vi "KeyBdReader.vi"(8 "error in (no error)":errorcluster) -> (0 "error out":errorcluster)   [LabVIEW 2014]
uses:
  c_InstructionEnum.ctl
  g_Stop.vi
  <vilib>/Utility/inputDevices.llb/keyboardAcquire.vi
  g_CommandParam.vi
  <vilib>/Utility/inputDevices.llb/closeKeyboard.vi
  c_PlatePosEnum.ctl
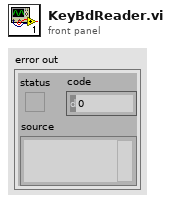
[diagram p1: front panel]
types:
  T1 = typedef "c_InstructionEnum.ctl" = enum16{"Move Absolute", "Increment", "Move Home", "Motion Kill", "Move Plate", "Set Stepsize", "Query Position"}
  T2 = typedef "c_PlatePosEnum.ctl" = enum16{"Contact", "Seperate"}
  T3 = enum16{"0", "1", "2", "3", "4", "5", "6", "7", "8", "9", "A", "B", "C", "D", "E", "F", "G", "H", "I", "J", "K", "L", "M", "N", "O", "P", "Q", "R", "S", "T", "U", "V", "W", "X", "Y", "Z", "F1", "F2", "F3", "F4", "F5", "F6", "F7", "F8", "F9", "F10", "F11", "F12", "F13", "F14", "F15", "ADD", "BACK", "BACKSLASH", "CAPITAL", "COMMA", "DECIMAL", "DELETE", "DIVIDE", "DOWN", "END", "EQUALS", "ESCAPE", "GRAVE (`)", "HOME", "INSERT", "LBRACKET", "LCONTROL", "LEFT", "L ALT", "LSHIFT", "LWIN", "MINUS", "MULTIPLY", "NEXT", "NUMLOCK", "NUMPAD_0", "NUMPAD_1", "NUMPAD_2", "NUMPAD_3", "NUMPAD_4", "NUMPAD_5", "NUMPAD_6", "NUMPAD_7", "NUMPAD_8", "NUMPAD_9", "PAUSE", "PERIOD", "PRIOR (PG UP)", "RBRACKET", "RCONTROL", "RETURN", "RIGHT", "R ALT", "RSHIFT", "RWIN", "SCROLL", "SEMICOLON", "SLASH", "SPACE", "SUBTRACT", "TAB", "UP", "ENTER (num pad)", "' (quote)"}[]
  T4 = enum16{"0", "1", "2", "3", "4", "5", "6", "7", "8", "9", "A", "B", "C", "D", "E", "F", "G", "H", "I", "J", "K", "L", "M", "N", "O", "P", "Q", "R", "S", "T", "U", "V", "W", "X", "Y", "Z", "F1", "F2", "F3", "F4", "F5", "F6", "F7", "F8", "F9", "F10", "F11", "F12", "F13", "F14", "F15", "ADD", "BACK", "BACKSLASH", "CAPITAL", "COMMA", "DECIMAL", "DELETE", "DIVIDE", "DOWN", "END", "EQUALS", "ESCAPE", "GRAVE (`)", "HOME", "INSERT", "LBRACKET", "LCONTROL", "LEFT", "L ALT", "LSHIFT", "LWIN", "MINUS", "MULTIPLY", "NEXT", "NUMLOCK", "NUMPAD_0", "NUMPAD_1", "NUMPAD_2", "NUMPAD_3", "NUMPAD_4", "NUMPAD_5", "NUMPAD_6", "NUMPAD_7", "NUMPAD_8", "NUMPAD_9", "PAUSE", "PERIOD", "PRIOR (PG UP)", "RBRACKET", "RCONTROL", "RETURN", "RIGHT", "R ALT", "RSHIFT", "RWIN", "SCROLL", "SEMICOLON", "SLASH", "SPACE", "SUBTRACT", "TAB", "UP", "ENTER (num pad)", "' (quote)"}
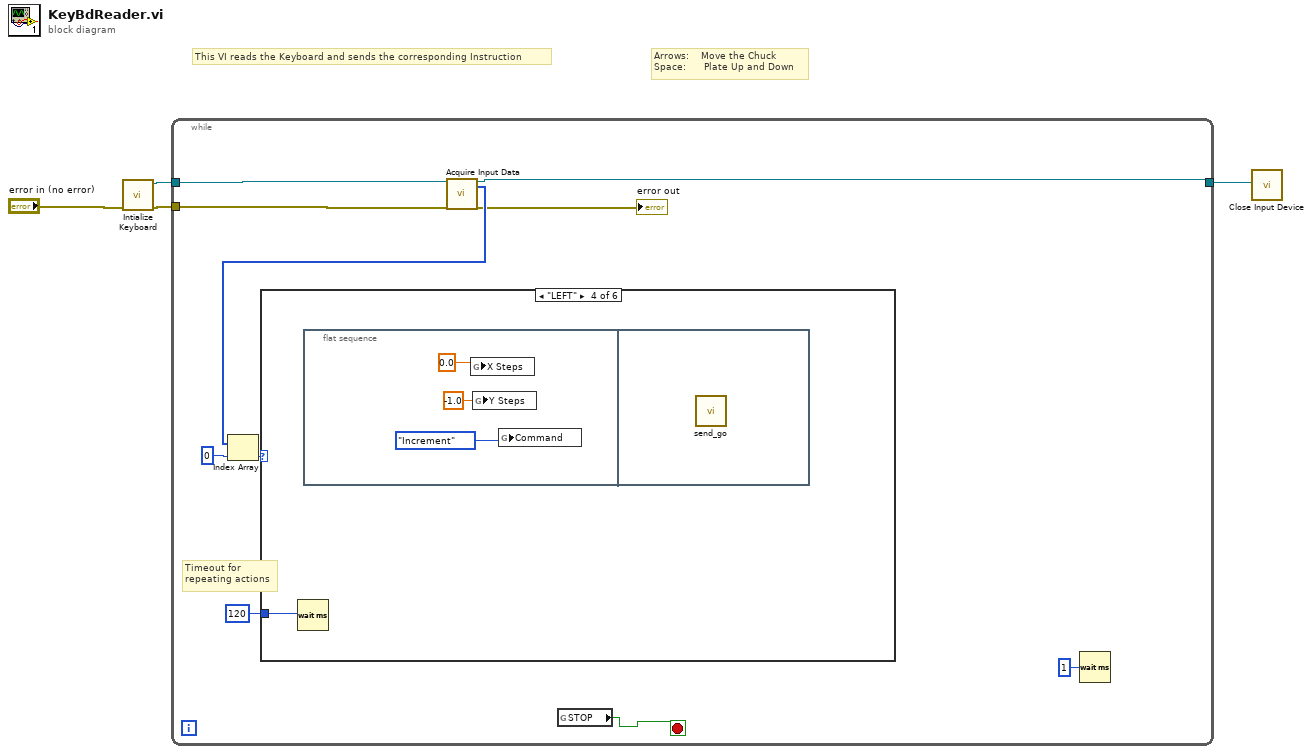
[diagram p0: block diagram]
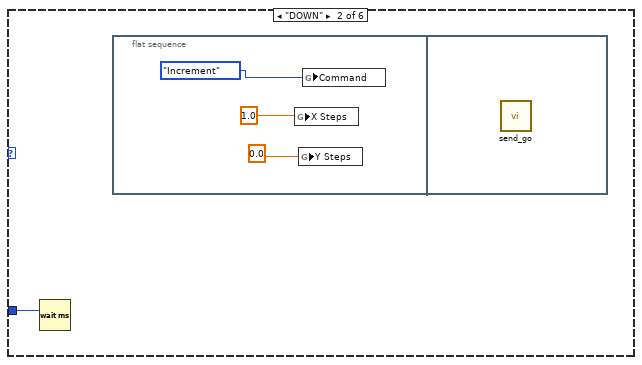
[diagram p3: hidden frame]
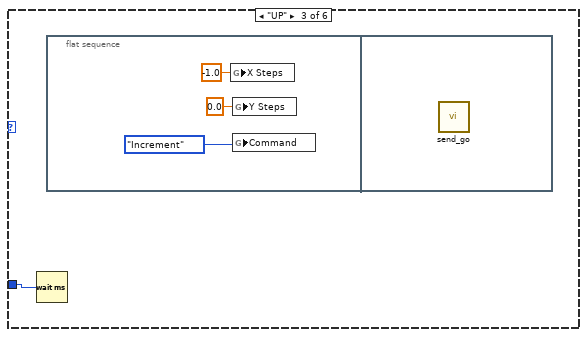
[diagram p4: hidden frame]
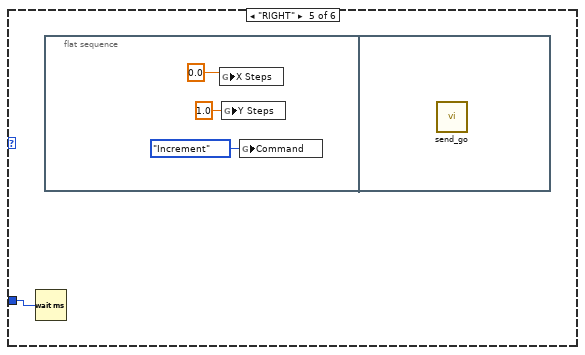
[diagram p5: hidden frame]
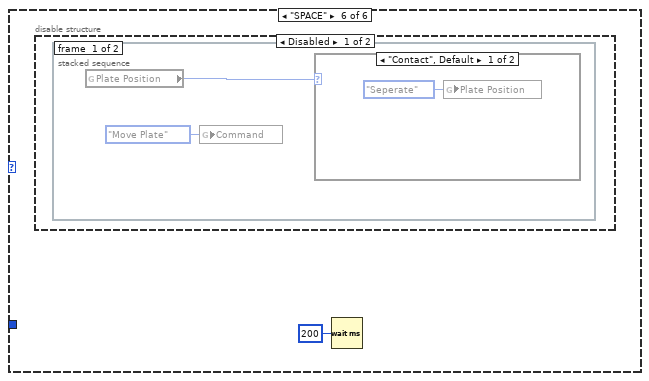
[diagram p6: hidden frame]
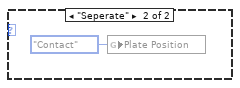
[diagram p7: hidden frame]
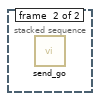
[diagram p8: hidden frame]
diagram:
  # "Arrows:    Move the Chuck\nSpace:      Plate Up and Down"
  # "This VI reads the Keyboard and sends the corresponding Instruction"
  n1 = call <vilib>:"Intialize Keyboard.vi"("error in (no error)"="error in (no error)") -> ("error out"=w3:errorcluster, "device ID"=w2:refnum<k1>)  [unwired: 9 in]
  n2 = while {
    tunnel: w3 -> [w14]
    tunnel: w2 -> [w13]
    tunnel: [w12] -> w1
    stop <- w8 stop-if-true
    # "Timeout for \nrepeating actions"
    n3 = call-poly <vilib>:"Acquire Input Data.vi"("device ID"=w13, "error in (no error)"=w14) -> ("device ID"=w12:refnum<k1>, "keys pressed"=w10:T3, "error out"=→"error out":errorcluster)  [unwired: 15 in]
    n4 = Index Array(array=w10, index=0) -> (element=w9:T4)
    n5 = case shown="\"LEFT\"" w9 {
      tunnel: 120 -> [_ w15 w19 w23 w27 _]
      frame Default {
      }
      frame "DOWN" {
        n6 = Wait (ms)(milliseconds to wait=w15) -> ()  [unwired: 1 out]
        n7 = flat-sequence {
          frame #0 {
            n8 = global write "g_CommandParam.vi" "X Steps"(1.0 ("X Steps")) -> ()
            n9 = global write "g_CommandParam.vi" "Y Steps"(0.0 ("Y Steps")) -> ()
            n10 = global write "g_CommandParam.vi" "Command"(c_InstructionEnum."Increment" ("Command")) -> ()
          }
          frame #1 {
            n11 = call "send_go.vi"() -> ()  [unwired: 12 in]
          }
        }
      }
      frame "UP" {
        n12 = Wait (ms)(milliseconds to wait=w19) -> ()  [unwired: 1 out]
        n13 = flat-sequence {
          frame #0 {
            n14 = global write "g_CommandParam.vi" "X Steps"(-1.0 ("X Steps")) -> ()
            n15 = global write "g_CommandParam.vi" "Y Steps"(0.0 ("Y Steps")) -> ()
            n16 = global write "g_CommandParam.vi" "Command"(c_InstructionEnum."Increment" ("Command")) -> ()
          }
          frame #1 {
            n17 = call "send_go.vi"() -> ()  [unwired: 12 in]
          }
        }
      }
      frame "LEFT" {
        n18 = Wait (ms)(milliseconds to wait=w23) -> ()  [unwired: 1 out]
        n19 = flat-sequence {
          frame #0 {
            n20 = global write "g_CommandParam.vi" "X Steps"(0.0 ("X Steps")) -> ()
            n21 = global write "g_CommandParam.vi" "Y Steps"(-1.0 ("Y Steps")) -> ()
            n22 = global write "g_CommandParam.vi" "Command"(c_InstructionEnum."Increment" ("Command")) -> ()
          }
          frame #1 {
            n23 = call "send_go.vi"() -> ()  [unwired: 12 in]
          }
        }
      }
      frame "RIGHT" {
        n24 = Wait (ms)(milliseconds to wait=w27) -> ()  [unwired: 1 out]
        n25 = flat-sequence {
          frame #0 {
            n26 = global write "g_CommandParam.vi" "X Steps"(0.0 ("X Steps")) -> ()
            n27 = global write "g_CommandParam.vi" "Y Steps"(1.0 ("Y Steps")) -> ()
            n28 = global write "g_CommandParam.vi" "Command"(c_InstructionEnum."Increment" ("Command")) -> ()
          }
          frame #1 {
            n29 = call "send_go.vi"() -> ()  [unwired: 12 in]
          }
        }
      }
      frame "SPACE" {
        n30 = disable-structure shown="Disabled" {
          frame Disabled {
            n31 = stacked-sequence {
              frame #0 {
                n32 = global read "g_CommandParam.vi" "Plate Position"() -> (w33:T2)
                n33 = global write "g_CommandParam.vi" "Command"(c_InstructionEnum."Move Plate" ("Command")) -> ()
                n34 = case shown="\"Contact\", Default" w33 {
                  frame "Contact", Default {
                    n35 = global write "g_CommandParam.vi" "Plate Position"(c_PlatePosEnum."Seperate" ("Plate Position")) -> ()
                  }
                  frame "Seperate" {
                    n36 = global write "g_CommandParam.vi" "Plate Position"(c_PlatePosEnum."Contact" ("Plate Position")) -> ()
                  }
                }
              }
              frame #1 {
                n37 = call "send_go.vi"() -> ()  [unwired: 12 in]
              }
            }
          }
          frame Enabled {
          }
        }
        n38 = Wait (ms)(milliseconds to wait=u32 200) -> ()  [unwired: 1 out]
      }
    }
    n39 = global read "g_Stop.vi" "STOP"() -> (w8:bool)
    n40 = Wait (ms)(milliseconds to wait=u32 1) -> ()  [unwired: 1 out]
  }
  n41 = call-poly <vilib>:"Close Input Device.vi"("device ID"=w1) -> ()  [unwired: 9 in, 1 out]
